vi "Get Type.vi"(11 "Timestamp in":refnum<class "Timestamp.lvclass">) -> (3 "Type":string)   [LabVIEW 2019, in "Timestamp.lvclass"]
uses:
  <vilib>/gpm_packages/@cs/data-type-serializer/source/Timestamp/Timestamp.lvclass
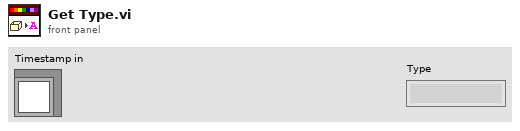
[diagram p1: front panel]
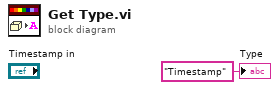
[diagram p0: block diagram]
diagram:
  "Type" <- "Timestamp" ("Type")
